vi "Get No Valid Step Values.vi"(8 "error in (no error)":errorcluster, 11 "Output Sequencer in":refnum<class "Output Sequencer.lvclass">) -> (0 "error out":errorcluster, 1 "Digital Values to Write":bool[](array[boolean]), 2 "Analog Values to Write":dbl[](array[numeric]), 3 "Output Sequencer out":refnum<class "Output Sequencer.lvclass">)   [LabVIEW 2020, in "Output Sequencer.lvlib" / "Output Sequencer.lvclass"]
uses:
  Output Sequencer.lvclass
  Output Sequencer.lvclass/Output Sequencer.ctl
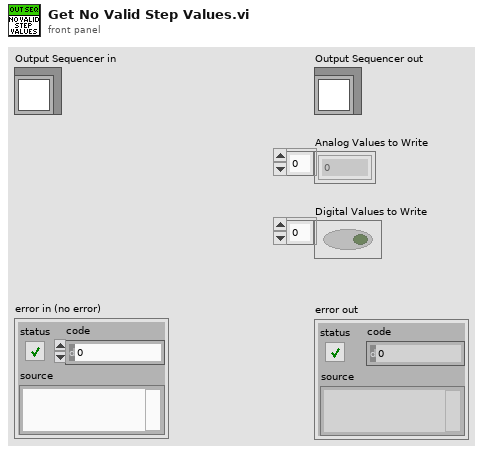
[diagram p1: front panel]
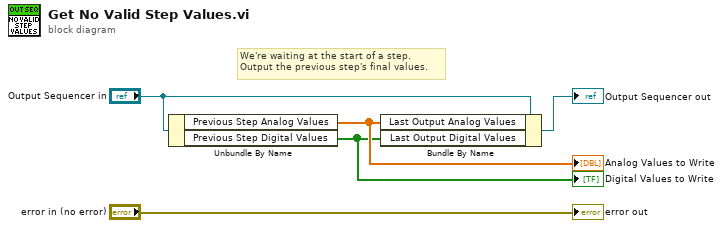
[diagram p0: block diagram]
diagram:
  # "We're waiting at the start of a step.\nOutput the previous step's final values."
  n1 = Unbundle By Name("Output Sequencer in") -> ("Previous Step Analog Values"=w3:dbl[], "Previous Step Digital Values"=w2:bool[])
  "Digital Values to Write" <- w2
  "Analog Values to Write" <- w3
  n2 = Bundle By Name(cluster="Output Sequencer in", "Last Output Analog Values"=w3, "Last Output Digital Values"=w2) -> (→"Output Sequencer out":refnum<class "Output Sequencer.lvclass">)
  "error out" <- "error in (no error)"
